vi "Read Number of Words and Parameters.vi"(8 "error in":errorcluster, 11 "message ref in":refnum<k20>) -> (0 "error out":errorcluster, 1 "parameters":T2(array[cluster]), 2 "number of words":u16, 3 "message ref out":refnum<k20>)   [LabVIEW 2020, in "AIM MIL-STD 1553 Import.lvlib"]
uses:
  AIM MIL-STD 1553 Import.lvlib
  15af4859-c171-48a8-8352-729fb2fbacc4.vi
  Constants.vi
  Shared/Parameter Definition.ctl
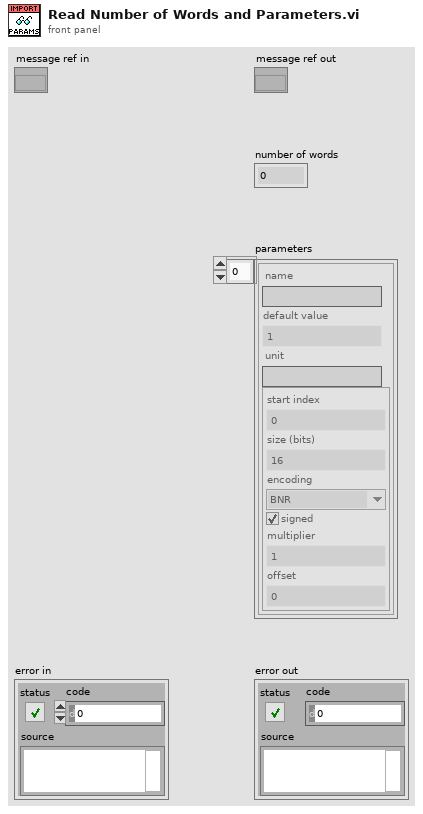
[diagram p1: front panel]
types:
  T1 = typedef "Parameter Definition.ctl" = cluster{"start index":i32, "size (bits)":i32, "encoding":enum16{"BNR", "BCD", "Discrete"}, "signed":bool, "multiplier":dbl, "offset":dbl}
  T2 = cluster{"name":string, "default value":dbl, "unit":string, "parameter definition":T1}[]
  T3 = cluster{"name":string, "default value":dbl, "unit":string, "parameter definition":T1}
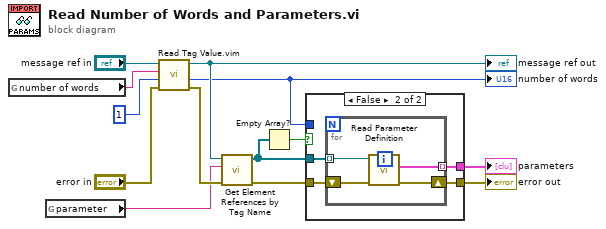
[diagram p0: block diagram]
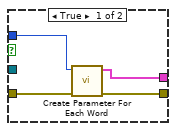
[diagram p2: hidden frame]
diagram:
  n1 = global read "Constants.vi" "number of words"() -> (w13:string)
  n2 = global read "Constants.vi" "parameter"() -> (w2:string)
  n3 = call "Read Tag Value.vim"("error in"="error in", "default"=u16 1, "tag name"=w13, "node in"="message ref in") -> ("error out"=w8:errorcluster, "value"=w6:u16, "node out"=w9:refnum<k20>)  [unwired: 5 in]
  "number of words" <- w6
  "message ref out" <- w9
  n4 = call "Get Element References by Tag Name.vi"("error in"=w8, "tag name"=w2, "node in"=w9) -> ("error out"=w4:errorcluster, "array of elements"=w1:refnum<k20>[])  [unwired: 7 in]
  n5 = Empty Array?(array=w1) -> (empty?=w7:bool)
  n6 = case shown="False" w7 {
    tunnel: w6 -> [w17 _]
    tunnel: [w16 w21] -> w5
    tunnel: w4 -> [w15 w20]
    tunnel: [w14 w19] -> w3
    tunnel: w1 -> [_ w18]
    frame True {
      n7 = call "Create Parameter For Each Word.vi"("error in"=w15, "number of words"=w17) -> ("error out"=w14:errorcluster, "parameters"=w16:T2)  [unwired: 8 in]
    }
    frame False {
      n8 = for {
        tunnel: [w22] -> w21 mode=indexing
        shift-right: [w24] -> w19
        shift-left: w20 -> [w25]
        tunnel: w18 -> [w23] mode=indexing
        n9 = call "Read Parameter Definition.vi"("error in"=w25, "parameter ref in"=w23) -> ("error out"=w24:errorcluster, "parameter"=w22:T3)  [unwired: 7 in, 1 out]
      }
    }
  }
  "error out" <- w3
  "parameters" <- w5
